vi "closeLog.vi"(8 "error in (no error)":errorcluster, 11 "Model in":refnum<class "Model.lvclass">) -> (0 "error out":errorcluster, 3 "Model out":refnum<class "Model.lvclass">)   [LabVIEW 2013, in "Model.lvclass"]
uses:
  Model.lvclass
  Model.lvclass/Model.ctl
  <userlib>/Common/Log/Log/Log.lvclass
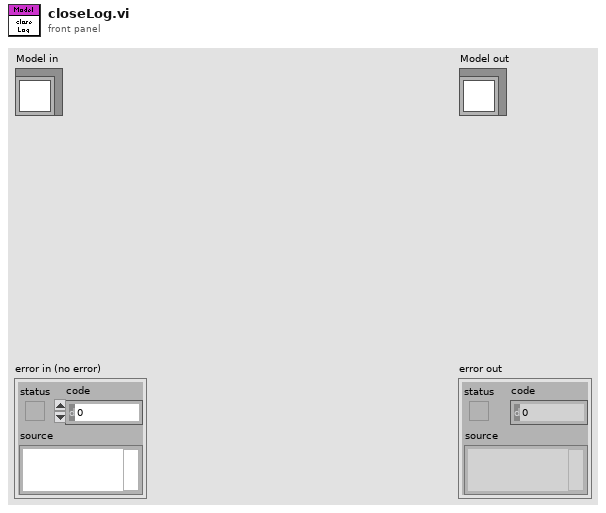
[diagram p1: front panel]
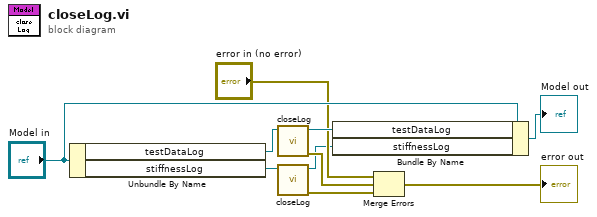
[diagram p0: block diagram]
diagram:
  n1 = Unbundle By Name("Model in") -> ("testDataLog"=w9:refnum<class "TestDataLog.lvclass">, "stiffnessLog"=w3:refnum<class "StiffnessLog.lvclass">)
  n2 = call <userlib>:"closeLog.vi"("Logger in"=w9) -> ("error out"=w5:errorcluster, "Logger out"=w8:refnum<class "TestDataLog.lvclass">)  [unwired: 9 in]
  n3 = call <userlib>:"closeLog.vi"("Logger in"=w3) -> ("error out"=w1:errorcluster, "Logger out"=w2:refnum<class "StiffnessLog.lvclass">)  [unwired: 9 in]
  n4 = Bundle By Name(cluster="Model in", "testDataLog"=w8, "stiffnessLog"=w2) -> (→"Model out":refnum<class "Model.lvclass">)
  n5 = Merge Errors("error in (no error)", w5, w1) -> (→"error out":errorcluster)
